vi "NI stop task.vi"(8 "error in (no error)":errorcluster, 11 "NI in":refnum<class "NI.lvclass">) -> (0 "error out":errorcluster, 3 "NI out":refnum<class "NI.lvclass">)   [LabVIEW 2021, in "NI.lvlib" / "NI.lvclass"]
uses:
  NI.lvclass
  C:/Program Files (x86)/National Instruments/LabVIEW 2021/vi.lib/ActorFramework/Actor/Actor.lvclass
  NI.lvclass/NI.ctl
  Main_Control/Main_Control/notifications.ctl
  <vilib>/ActorFramework/Actor/Actor.lvclass/Actor.ctl
  Main_Control/Main_Control Messages/UI notifier Msg/UI notifier Msg.lvclass/UI notifier Msg.ctl
  <vilib>/ActorFramework/Message Enqueuer/Message Enqueuer.lvclass/Message Enqueuer.ctl
  <vilib>/ActorFramework/Message Enqueuer/Enqueue.vi
  Main_Control/Main_Control Messages/UI notifier Msg/UI notifier Msg.lvclass
  C:/Program Files (x86)/National Instruments/LabVIEW 2021/vi.lib/ActorFramework/Message/Message.lvclass
  <vilib>/ActorFramework/Message Priority Queue/Priority Enqueue.vi
  <vilib>/DAQmx/write.llb/DAQmx Write (Analog 1D DBL NChan 1Samp).vi
  <vilib>/ActorFramework/Actor/Actor.lvclass
  Main_Control/Main_Control/Main_Control.lvclass
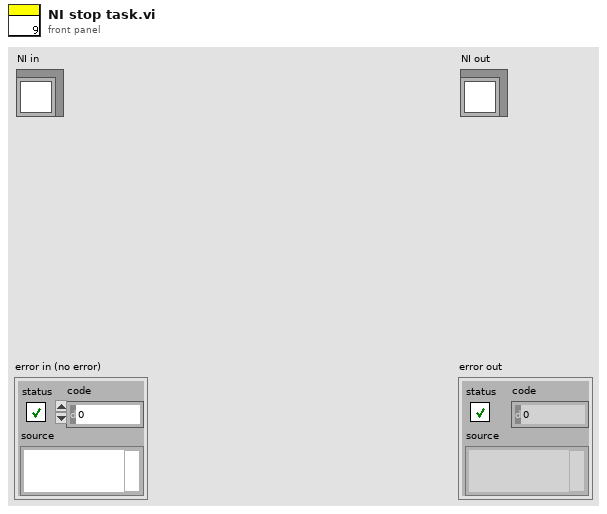
[diagram p1: front panel]
types:
  T1 = typedef "Main_Control.lvlib/Main_Control.lvclass/notifications.ctl" = enum16{"cam 1 frame skkipped", "cam finish", "cam started", "cam stopped", "cam updated", "ni started", "ni stopped", "ni updated"}
  T2 = cluster{"AO1 laser":refnum<k21>, "AO2 zy":refnum<k21>, "CO1 mainTrig":refnum<k21>, "CO2 fastClock":refnum<k21>, "AI phase":refnum<k21>}
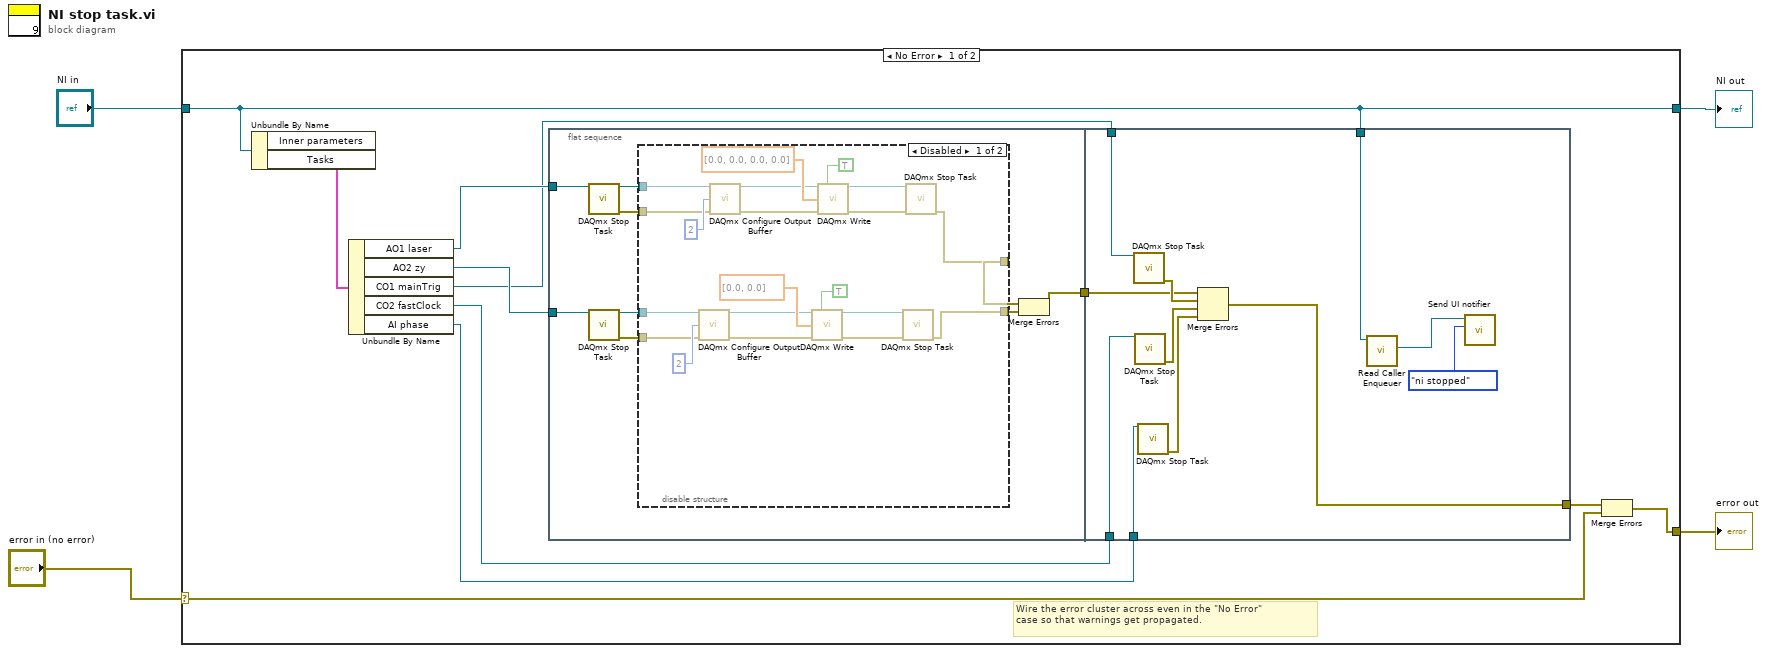
[diagram p0: block diagram]
diagram:
  n1 = case shown="No Error" "error in (no error)" {
    selector: "error in (no error)" -> [w8 w59]
    tunnel: [w7 w59] -> w3
    tunnel: [w5 w58] -> w1
    tunnel: "NI in" -> [w5 w58]
    frame No Error {
      # "Wire the error cluster across even in the \"No Error\"\ncase so that warnings get propagated."
      n2 = Unbundle By Name(w5) -> ("Tasks"=w15:T2)  [unwired: 1 out]
      n3 = Unbundle By Name(w15) -> ("AO1 laser"=w14:refnum<k21>, "AO2 zy"=w13:refnum<k21>, "CO1 mainTrig"=w12:refnum<k21>, "CO2 fastClock"=w11:refnum<k21>, "AI phase"=w10:refnum<k21>)
      n4 = flat-sequence {
        tunnel: w14 -> [w18]
        tunnel: w13 -> [w24]
        tunnel: [w21] -> w9
        tunnel: [w57] -> w6
        tunnel: w5 -> [w56]
        tunnel: w9 -> [w49]
        tunnel: w10 -> [w51]
        tunnel: w11 -> [w55]
        tunnel: w12 -> [w54]
        frame #0 {
          n5 = call <vilib>:"DAQmx Stop Task.vi"("task/channels in"=w18) -> ("task out"=w17:refnum<k21>, "error out"=w16:errorcluster)  [unwired: 13 in]
          n6 = call <vilib>:"DAQmx Stop Task.vi"("task/channels in"=w24) -> ("task out"=w20:refnum<k21>, "error out"=w19:errorcluster)  [unwired: 13 in]
          n7 = disable-structure shown="Disabled" {
            disable-tunnel: w18 -> [_ _]
            disable-tunnel: [w40 w46] -> w23
            disable-tunnel: [w39 w45] -> w22
            disable-tunnel: w20 -> [w34 _]
            disable-tunnel: w19 -> [w33 w45]
            disable-tunnel: w17 -> [w26 _]
            disable-tunnel: w16 -> [w25 w46]
            frame Disabled {
              n8 = call <vilib>:"DAQmx Configure Output Buffer.vi"("task/channels in"=w34, "buffer size (in samples per channel)"=u32 2, "error in"=w33) -> ("task out"=w31:refnum<k21>, "error out"=w32:errorcluster)  [unwired: 11 in]
              n9 = call <vilib>:"DAQmx Configure Output Buffer.vi"("task/channels in"=w26, "buffer size (in samples per channel)"=u32 2, "error in"=w25) -> ("task out"=w37:refnum<k21>, "error out"=w36:errorcluster)  [unwired: 11 in]
              n10 = call-poly <vilib>:"DAQmx Write.vi"("task/channels in"=w31, "auto start"=TRUE, "data"=dbl[] [0.0, 0.0], "error in"=w32) -> ("task out"=w30:refnum<k21>, "error out"=w29:errorcluster)  [unwired: 9 in, 1 out]
              n11 = call-poly <vilib>:"DAQmx Write.vi"("task/channels in"=w37, "auto start"=TRUE, "data"=dbl[] [0.0, 0.0, 0.0, 0.0], "error in"=w36) -> ("task out"=w28:refnum<k21>, "error out"=w27:errorcluster)  [unwired: 9 in, 1 out]
              n12 = call <vilib>:"DAQmx Stop Task.vi"("task/channels in"=w30, "error in"=w29) -> ("error out"=w39:errorcluster)  [unwired: 12 in, 1 out]
              n13 = call <vilib>:"DAQmx Stop Task.vi"("task/channels in"=w28, "error in"=w27) -> ("error out"=w40:errorcluster)  [unwired: 12 in, 1 out]
            }
            frame Enabled {
              # "dont know how to elegantly\nset laser and galvo to off after task done"
            }
          }
          n14 = Merge Errors(w23, w22) -> (w21:errorcluster)
        }
        frame #1 {
          n15 = call <vilib>:"DAQmx Stop Task.vi"("task/channels in"=w54) -> ("error out"=w53:errorcluster)  [unwired: 13 in, 1 out]
          n16 = call <vilib>:"DAQmx Stop Task.vi"("task/channels in"=w55) -> ("error out"=w52:errorcluster)  [unwired: 13 in, 1 out]
          n17 = call <vilib>:"DAQmx Stop Task.vi"("task/channels in"=w51) -> ("error out"=w50:errorcluster)  [unwired: 13 in, 1 out]
          n18 = Merge Errors(w49, w53, w52, w50) -> (w57:errorcluster)
          n19 = call <vilib>:"Read Caller Enqueuer.vi"("Actor"=w56) -> ("Caller Enqueuer"=w47:refnum<class "Message Enqueuer.lvclass">)  [unwired: 10 in]
          n20 = call "Send UI notifier.vi"("Object&State"=notifications."ni stopped", "Message Enqueuer"=w47) -> ()  [unwired: 8 in, 2 out]
        }
      }
      n21 = Merge Errors(w6, w8) -> (w7:errorcluster)
    }
    frame Error {
    }
  }
  "error out" <- w3
  "NI out" <- w1
